vi "Adam_Puff.vi"() -> (5 "Plug in titles":string[](array[string]), 7 "Plug in values":string[](array[string]))   [LabVIEW 2014]
uses:
  Controls/Setup.ctl
  Controls/Post_Process.ctl
  Globals/Meas_global.vi
panel:
  in  "Initial bkgnd Sec":u32=30
  in  "Seconds to measure":dbl=800.0
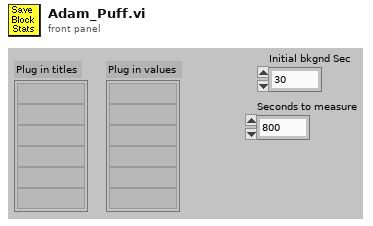
[diagram p1: front panel]
types:
  T1 = typedef "Post_Process.ctl" = enum16{"Take New Data", "Post Process Raw Data File"}
  T2 = typedef "Setup.ctl" = enum16{"Run Program", "Show Setup", "Save Current Setup", "Setup Front Panel"}
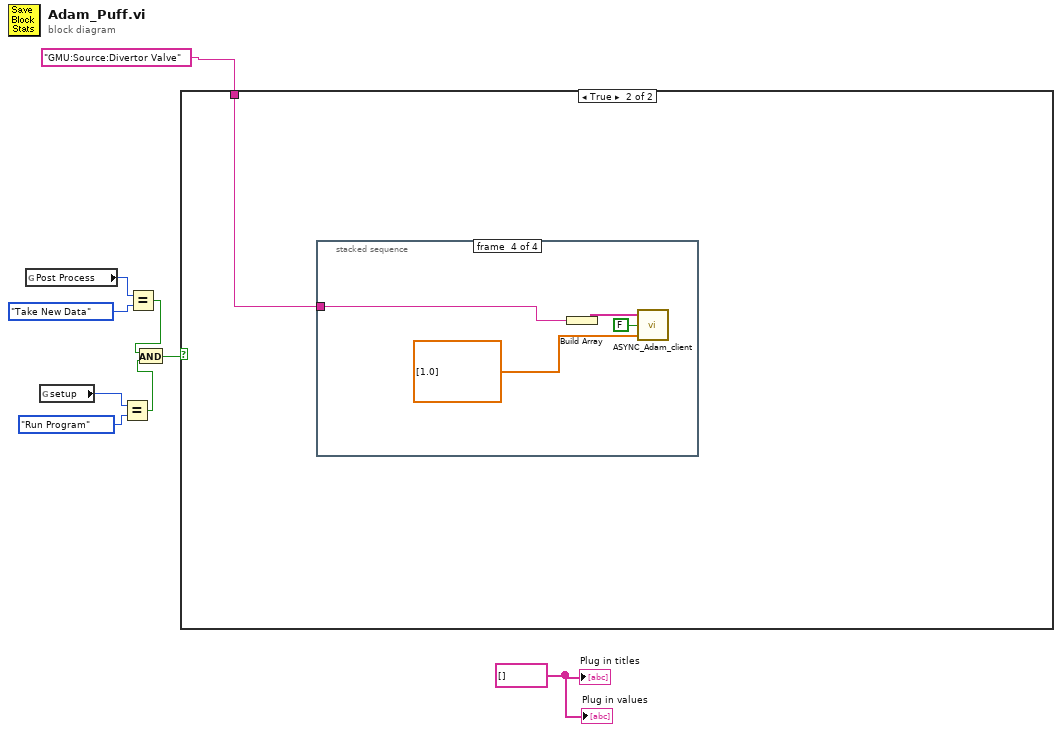
[diagram p0: block diagram]
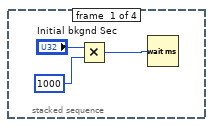
[diagram p3: hidden frame]
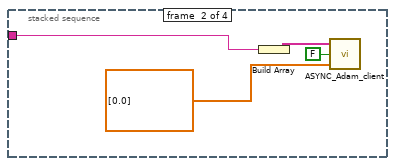
[diagram p4: hidden frame]
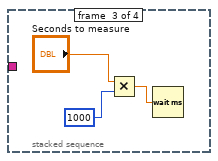
[diagram p5: hidden frame]
diagram:
  w9 = string[] [] ("Plug in titles")
  n1 = global read "Meas_global.vi" "Post Process"() -> (w7:T1)
  n2 = global read "Meas_global.vi" "setup"() -> (w6:T2)
  n3 = Equal?(x=w6, y=Setup."Run Program" ("setup")) -> (x = y?=w4:bool)
  n4 = Equal?(x=w7, y=Post_Process."Take New Data" ("Post Process")) -> (x = y?=w3:bool)
  n5 = And(x=w3, y=w4) -> (x .and. y?=w2:bool)
  n6 = case shown="True" w2 {
    tunnel: "GMU:Source:Divertor Valve" -> [_ w10]
    frame False {
    }
    frame True {
      n7 = stacked-sequence {
        tunnel: w10 -> [_ w15 _ w22]
        frame #0 {
          n8 = Multiply(x="Initial bkgnd Sec", y=u32 1000 ("milliseconds to wait")) -> (x*y=w11:u32)
          n9 = Wait (ms)(milliseconds to wait=w11) -> ()  [unwired: 1 out]
        }
        frame #1 {
          n10 = Build Array(w15) -> (w17:string[])
          n11 = call "ASYNC_Adam_client.vi"("Values"=dbl[] [0.0], "Check Value is in the scan table?"=FALSE, "Channel Names"=w17) -> ()  [unwired: 2 out]
        }
        frame #2 {
          n12 = Multiply(x="Seconds to measure", y=u32 1000 ("milliseconds to wait")) -> (x*y=w18:dbl)
          n13 = Wait (ms)(milliseconds to wait=w18) -> ()  [unwired: 1 out]
        }
        frame #3 {
          n14 = Build Array(w22) -> (w24:string[])
          n15 = call "ASYNC_Adam_client.vi"("Values"=dbl[] [1.0], "Check Value is in the scan table?"=FALSE, "Channel Names"=w24) -> ()  [unwired: 2 out]
        }
      }
    }
  }
  "Plug in values" <- w9
  "Plug in titles" <- w9
